vi "ReadObjectLayout.vi"(7 "properties to ignore":variant, 8 "error in (no error)":errorcluster, 10 "GObj Refnum":refnum<vi>, 11 "Tab Control Layout in":refnum<class "Tab Control Layout.lvclass">) -> (0 "error out":errorcluster, 3 "Tab Control Layout out":refnum<class "Tab Control Layout.lvclass">)   [LabVIEW 2012, in "NI_SE_Front Panel Layout.lvlib" / "Tab Control Layout.lvclass"]
doc: "Read layout information from the GObj Refnum."
uses:
  Tab Control Layout.lvclass
  Object Layout/Object Layout.lvclass
  Tab Control Layout.lvclass/Tab Control Layout.ctl
  Control Layout/Control Layout.lvclass
  NI_SE_Front Panel Layout.lvlib
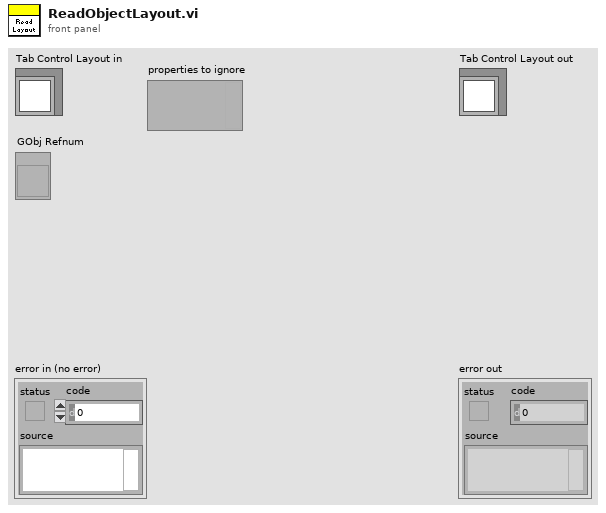
[diagram p1: front panel]
types:
  T1 = typedef "LVBoundsTypeDef.ctl" = cluster{"Width":u32, "Height":u32}
  T2 = enum32{"Size Tabs To Contents", "Size All Tabs to Largest Tab", "Fixed Tab Size"}
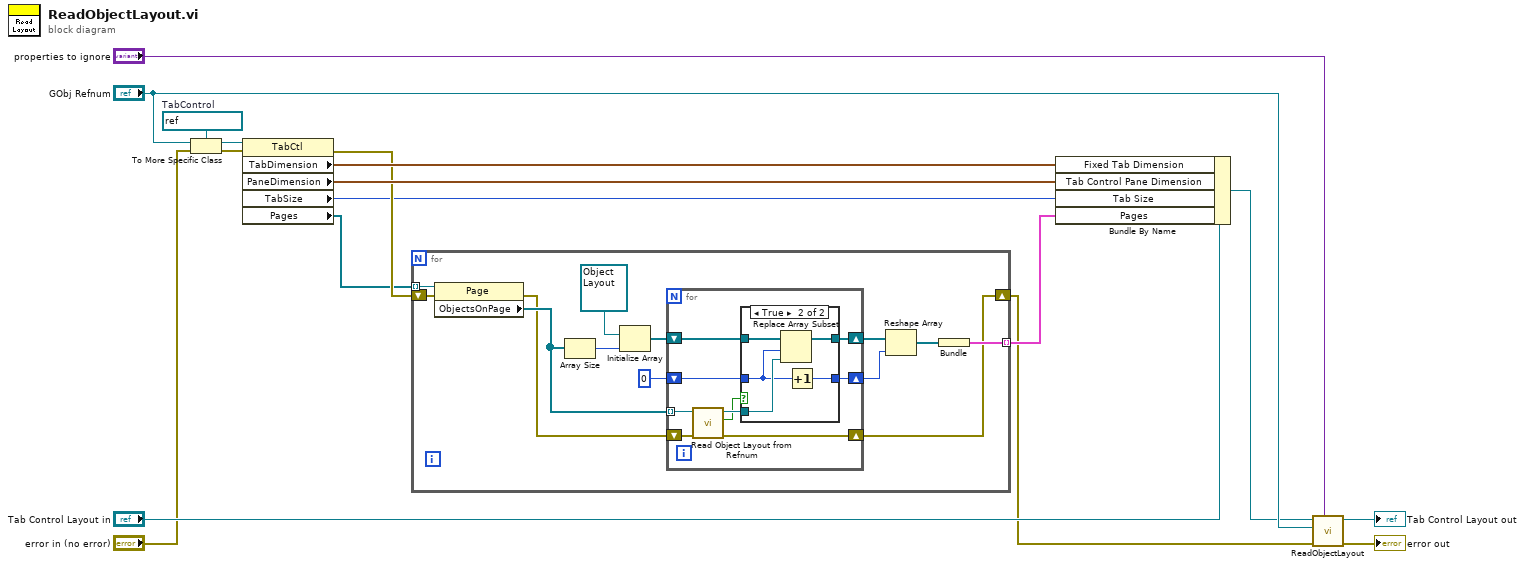
[diagram p0: block diagram]
diagram:
  w10 = refnum<vi> refnum  # TabControl
  n1 = To More Specific Class(target class=w10, reference="GObj Refnum", error in="error in (no error)") -> (specific class reference=w9:refnum<vi>, error out=w8:errorcluster)
  n2 = property class="TabCtl"(reference=w9, error in=w8) -> (error out=w5:errorcluster, "TabDimension"=w7:T1, "PaneDimension"=w6:T1, "TabSize"=w3:T2, "Pages"=w4:refnum<vi>[])  [unwired: 1 out]
  n3 = for {
    tunnel: w4 -> [w30] mode=indexing
    shift-right: [w18] -> w1
    shift-left: w5 -> [w29]
    tunnel: [w19] -> w2 mode=indexing
    n4 = property class="Page"(reference=w30, error in=w29) -> (error out=w21:errorcluster, "ObjectsOnPage"=w22:refnum<vi>[])  [unwired: 1 out]
    n5 = Array Size(array=w22) -> (size(s)=w24:i32)
    n6 = Initialize Array(refnum<class "Object Layout.lvclass"> refnum ("object layout"), w24) -> (w25:refnum<class "Object Layout.lvclass">[])
    n7 = for {
      tunnel: w22 -> [w39] mode=indexing
      shift-right: [w36] -> w18
      shift-left: w21 -> [w37]
      shift-right: [w33] -> w27
      shift-left: w25 -> [w34]
      shift-right: [w31] -> w28
      shift-left: 0 -> [w32]
      n8 = call "Read Object Layout from Refnum.vi"("error in"=w37, "GObj refnum"=w39) -> ("error out"=w36:errorcluster, "found?"=w35:bool, "object layout"=w38:refnum<class "Object Layout.lvclass">)  [unwired: 7 in]
      n9 = case shown="True" w35 {
        tunnel: w34 -> [w41 w46]
        tunnel: w38 -> [_ w45]
        tunnel: [w41 w44] -> w33
        tunnel: w32 -> [w40 w43]
        tunnel: [w40 w42] -> w31
        frame False {
        }
        frame True {
          n10 = Replace Array Subset(array=w46, new element=w45, index=w43) -> (w44:refnum<class "Object Layout.lvclass">[])
          n11 = Increment(x=w43) -> (x+1=w42:i32)
        }
      }
    }
    n12 = Reshape Array(w27, w28) -> (w20:refnum<class "Object Layout.lvclass">[])
    n13 = Bundle(w20) -> (w19:cluster{refnum<class "Object Layout.lvclass">[]})  [unwired: 1 in]
  }
  n14 = Bundle By Name(cluster="Tab Control Layout in", "Fixed Tab Dimension"=w7, "Tab Control Pane Dimension"=w6, "Tab Size"=w3, "Pages"=w2) -> (w14:refnum<class "Tab Control Layout.lvclass">)
  n15 = call-parent "ReadObjectLayout.vi"("properties to ignore"="properties to ignore", "error in (no error)"=w1, "GObj Refnum"="GObj Refnum", "Control Layout in"=w14) -> ("error out"=→"error out":errorcluster, "Control Layout out"=→"Tab Control Layout out":refnum<class "Tab Control Layout.lvclass">)  [unwired: 6 in]
